vi "Calculate number of miniscans.vi"(9 "XYZ Coordinates":T1[](array[typedef]) {"ROI group ID" format="%#_6f"; "Laser Power (%)" format="%#_6f"; "Zoom" format="%#_6f"; "Frame Size" format="%#_6f"; "Number of lines" format="%#_6f"; "Composite ID" format="%#_6f"; "Angle (deg)" format="%#_6f"; "ROI Time (ns)" format="%#_6f"; "ROI ID" format="%#_6f"; "Pixels in ROI" format="%#_6f"; "ROI index" format="%#_6f"; "Z stop" format="%#_6f"; "Y stop" format="%#_6f"; "X stop" format="%#_6f"; "Z start" format="%#_6f"; "X start" format="%#_6f"; "Y start" format="%#_6f"}, 11 "Acquisition length (sec)":dbl) -> (1 "Number of cycles":u64, 2 "Cycle time (us)":dbl, 3 "AOD fill time (us)":dbl)   [LabVIEW 2013]
uses:
  User Interface/Visualisation/Functional Imaging Viewer/Typedefs/ROI parameters data type.ctl
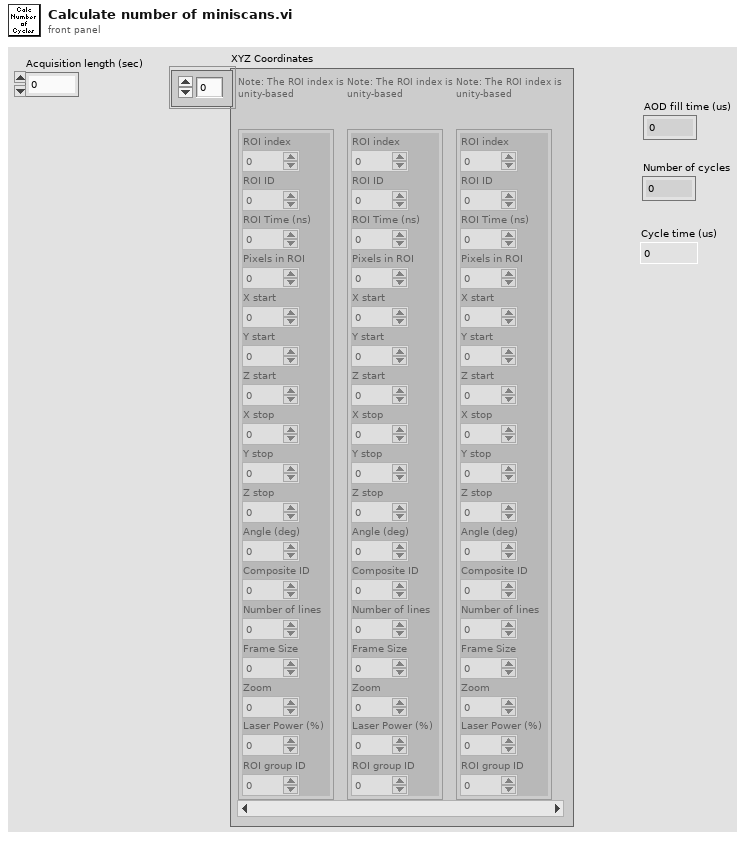
[diagram p1: front panel]
types:
  T1 = typedef "ROI parameters data type.ctl" = cluster{"ROI index":dbl, "ROI ID":dbl, "ROI Time (ns)":dbl, "Pixels in ROI":dbl, "X start":dbl, "Y start":dbl, "Z start":dbl, "X stop":dbl, "Y stop":dbl, "Z stop":dbl, "Angle (deg)":dbl, "Composite ID":dbl, "Number of lines":dbl, "Frame Size":dbl, "Zoom":dbl, "Laser Power (%)":dbl, "ROI group ID":dbl}
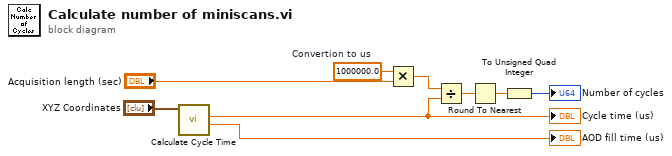
[diagram p0: block diagram]
diagram:
  w9 = 1000000.0  # Convertion to us
  n1 = call "Calculate Cycle Time.vi"("Coordinates"="XYZ Coordinates") -> ("AOD fill time (us)"=→"AOD fill time (us)":dbl, "Cycle time (us)"=w1:dbl)  [unwired: 9 in]
  "Cycle time (us)" <- w1
  n2 = Multiply(x=w9, y="Acquisition length (sec)") -> (x*y=w8:dbl)
  n3 = Divide(x=w8, y=w1) -> (x/y=w6:dbl)
  n4 = Round To Nearest(number=w6) -> (nearest integer value=w7:dbl)
  n5 = To Unsigned Quad Integer(1:w7) -> (0:→"Number of cycles":u64)
